vi "SYST_PRES.vi"(0 "VISA IN":refnum<visa-resource-name>, 5 "error in":errorcluster) -> (14 "VISA Out":refnum<visa-resource-name>, 19 "error out":errorcluster)   [LabVIEW 2018, in "PNA-X.lvlib"] (continued)
OFF (or 0) - Does NOT include DC Offset correction. \nExamples SENS:CORR:EXT:AUTO:DCOF 1 \nsense2:correction:extension:auto:dcoffset off \nQuery Syntax SENSe<cnum>:CORRection:EXTension:AUTO:DCOFfset? \nReturn Type Boolean \nDefault OFF (0) \nSENSe<cnum>:CORRection:EXTension:AUTO:LOSS <bool> \n(Read-Write) Specifies whether or not to include loss correction as part of automatic port extension. \nLearn more about Loss Compensation in port extension. \nParameters \n<cnum> Any existing channel number. If unspecified, value is set to 1 \n<bool> ON (or 1) - Includes Loss correction. \nOFF (or 0) - Does NOT include Loss correction. \nExamples SENS:CORR:EXT:AUTO:LOSS 1 \nsense2:correction:extension:auto:loss off \nQuery Syntax SENSe<cnum>:CORRection:EXTension:AUTO:LOSS? \nReturn Type Boolean \nDefault OFF (0) \nSENSe<cnum>:CORRection:EXTension:AUTO:MEASure <char> \n1701\n\n(Write-only) Measures either an OPEN or SHORT standard. When this command is sent, the PNA \nacquires the measurement with which to set automatic port extensions. Learn more about which \nstandard to measure. \nParameters \n<cnum> Any existing channel number. If unspecified, value is set to 1 \n<char> Standard to be measured. Choose from: \nOPEN Measure OPEN standard \nSHORt Measure SHORT standard \nExamples SENS:CORR:EXT:AUTO:MEAS OPEN \nsense2:correction:extension:auto:measure short \nQuery Syntax Not Applicable \nDefault Not Applicable \nSENSe<cnum>:CORRection:EXTension:AUTO:PORT<n> <bool> \n(Read-Write) Enables and disables automatic port extensions on the specified port. \nParameters \n<cnum> Any existing channel number. If unspecified, value is set to 1 \n<n> PNA Port number to enable or disable for automatic port extensions. \n<bool> ON (or 1) - Enable \nOFF (or 0) - Disable \nExamples SENS:CORR:EXT:AUTO:PORT2 0 \nsense2:correction:extension:auto:port4 on \nQuery Syntax SENSe<cnum>:CORRection:EXTension:AUTO:PORT<n>? \nReturn Type Boolean \nDefault All ports ON (enabled) \nSENSe<cnum>:CORRection:EXTension:AUTO:RESet \n1702\n\n(Write-only) Clears old port extension delay and loss data in preparation for acquiring new data. Send \nthis command prior to sending a new series of SENS:CORR:EXT:AUTO:MEAS. If acquiring both \nOPEN and SHORT standards, do not send this command between those acquisitions. \nParameters \n<cnum> Any existing channel number. If unspecified, value is set to 1 \nExamples SENS:CORR:EXT:AUTO:RES \nsense2:correction:extension:auto:reset \nQuery Syntax Not Applicable \nDefault Not Applicable \nSENSe<cnum>:CORRection:EXTension:AUTO:STARt <value> \n(Read-Write) Set the start frequency for custom user span. Learn more about User Span. \nParameters \n<cnum> Any existing channel number. If unspecified, value is set to 1 \n<value> User span start value. Must be within the frequency range of the active channel \nand less than the value set by SENS:CORR:EXT:AUTO:STOP. \nExamples SENS:CORR:EXT:AUTO:STAR 1E9 \nsense2:correction:extension:auto:start 200e6 \nQuery Syntax SENSe<cnum>:CORRection:EXTension:AUTO:STARt <value>? \nReturn Type Numeric \nDefault Start frequency of the current active channel. \nSENSe<cnum>:CORRection:EXTension:AUTO:STOP <value> \n1703\n\n(Read-Write) Set the stop frequency for custom user span. Learn more about User Span. \nParameters \n<cnum> Any existing channel number. If unspecified, value is set to 1 \n<value> User span stop value. Must be within the frequency range of the active channel \nand greater than the value set by SENS:CORR:EXT:AUTO:STARt \nExamples SENS:CORR:EXT:AUTO:STOP 1E9 \nsense2:correction:extension:auto:stop 200e6 \nQuery Syntax SENSe<cnum>:CORRection:EXTension:AUTO:STOP <value>? \nReturn Type Numeric \nDefault Stop frequency of the current active channel. \nSENSe<cnum>:CORRection:EXTension:PORT<pnum>:FREQ<n> <value> \n(Read-Write) Sets and returns the frequency \"Use\" number (1|2) for the specified port number. \nLearn about Loss Compensation values. \nParameters \n<cnum> Any existing channel number. If unspecified, value is set to 1 \n<pnum> Port Number that will receive the freq/loss settings. If unspecified, value is set \nto 1. \n<n> Frequency \"Use\" number. Choose from 1 or 2. If unspecified, value is set to 1. \n<value> Frequency value. Choose a frequency within the frequency span of the PNA. \nExamples SENS:CORR:EXT:PORT1:FREQ1 10E9 \nsense2:correction:extension:port2:freq2:2E10 \nQuery Syntax SENSe<cnum>:CORRection:EXTension:PORT<pnum>:FREQ<n>? \nReturn Type Numeric \nDefault 1 GHz \nSENSe<cnum>:CORRection:EXTension:PORT<pnum>:INCLude<n>:STATe <bool> \n1704\n\n(Read-Write) Sets and returns the ON/OFF state for the use of the Loss and Freq values for the \nspecified port number. \nLearn about Loss Compensation values. \nNote: This command affects ALL measurements on the specified channel. \nParameters \n<cnum> Any existing channel number. If unspecified, value is set to 1 \n<pnum> Port Number that will receive the Freq/Loss settings. If unspecified, value is set to \n1. \n<n> Freq and Loss pair. Choose from 1 or 2. If unspecified, value is set to 1. \n<value> State of Freq and Loss values for port extension. \n0 or OFF Specified Freq and Loss values are OFF \n1 or ON Specified Freq and Loss values are ON \nExamples SENS:CORR:EXT:PORT:INCL 0 \nsense2:correction:extension:port2:include:state on \nQuery Syntax SENSe<cnum>:CORRection:EXTension:PORT<pnum>:INCLude:STATe? \nReturn Type Boolean \nDefault OFF \nSENSe<cnum>:CORRection:EXTension:PORT<pnum>:LDC <value> \n(Read-Write) Sets and returns the Port Loss at DC value for the specified port number. \nLearn about Loss Compensation values. \nNote: This command affects ALL measurements on the specified channel. \nParameters \n<cnum> Any existing channel number. If unspecified, value is set to 1 \n<pnum> Port number to receive Loss value. If unspecified, value is set to 1. \n<value> Loss in dB. Choose a value between -90 and 90 \nExamples SENS:CORR:EXT:PORT:LDC 1.5 \nsense2:correction:extension:port2:ldc .1 \nQuery Syntax SENSe<cnum>:CORRection:EXTension:PORT<pnum>:LDC? \n1705\n\nReturn Type Numeric \nDefault 0 \nSENSe<cnum>:CORRection:EXTension:PORT<pnum>:LOSS<n> <value> \n(Read-Write) Sets and returns the Loss value for the specified port number. \nLearn about Loss Compensation values. \nNote: This command affects ALL measurements on the specified channel. \nParameters \n<cnum> Any existing channel number. If unspecified, value is set to 1 \n<pnum> Port Number that will receive the Freq/Loss settings. If unspecified, value is set \nto 1. \n<n> Loss \"Use\" number. Choose from 1 or 2. If unspecified, value is set to 1. \n<value> Loss in dB. Choose a value between -90 and 90 \nExamples SENS:CORR:EXT:PORT:LOSS1 1 \nsense2:correction:extension:port2:loss2 .1 \nQuery Syntax SENSe<cnum>:CORRection:EXTension:PORT<pnum>:LOSS<n>? \nReturn Type Numeric \nDefault 0 \nSENSe<cnum>:CORRection:EXTension:PORT<pnum>[:TIME] <num> \n1706\n\n(Read-Write) Sets the extension value at the specified port. Must also set SENS:CORR:EXT ON. \nNote: This command affects ALL measurements on the specified channel. \nParameters \n<cnum> Any existing channel number. If unspecified, value is set to 1 \n<pnum> Port Number that will receive the extension. If unspecified, value is set to 1. \n<num> The port extension in seconds; may include suffix. Choose a number between: \n-1E18 and 1E18 \nExamples SENS:CORR:EXT:PORT 2MS \nsense2:correction:extension:port2 .00025 \nQuery Syntax SENSe<cnum>:CORRection:EXTension:PORT<pnum> [:TIME]? \nReturn Type Numeric \nDefault 0 \nSENSe<cnum>:CORRection:EXTension:RECeiver<Rnum>[:TIME] <num> OBSOLETE \n(Read-Write) This command has NO replacement and no longer works. \nSets the extension value at the specified receiver. Must also set SENS:CORR:EXT ON. \nNote: Before using this command you must select a measurement using CALC:PAR:SEL. You can \nselect one measurement for each channel. \nParameters \n<cnum> Any existing channel number. If unspecified, value is set to 1 \n<Rnum> Number of the receiver that will receive the extension. If unspecified, value is \nset to 1 \nChoose from: \n1 for Receiver A \n2 for Receiver B \n<num> The electrical length in seconds; may include suffix. Choose a number \nbetween: \n-10 and 10 \nExamples SENS:CORR:EXT:REC 2MS \nsense2:correction:extension:receiver2:time .00025 \nQuery Syntax SENSe<cnum>:CORRection:EXTension:RECeiver<Rnum> [:TIME]? \n1707\n\nReturn Type Numeric \nDefault 0 \nSENSe<cnum>:CORRection:EXTension[:STATe] <ON | OFF> \n(Read-Write) Turns port extensions ON or OFF. \nParameters \n<cnum> Any existing channel number. If unspecified, value is set to 1 \n<ON | OFF> ON (or 1) - turns port extensions ON. \nOFF (or 0) - turns port extensions is OFF. \nExamples SENS:CORR:EXT ON \nsense2:correction:extension:state off \nQuery Syntax SENSe<cnum>:CORRection:EXTension[:STATe]? \nReturn Type Boolean (1 = ON, 0 = OFF) \nDefault OFF \n1708\n\nSense:Correction:Collect:Session Commands \nThe commands in this topic are common to perform both SMC and VMC calibrations. A calibration \nsession is a term used to describe an instance of a SMC or VMC calibration. For more commands, see \nSESS:SMC and SESS:VMC. \nCommands to read (STEP?) and describe (DESC?) each step are provided to facilitate a remote user \ninterface. \nTo perform a NON - SMC or VMC calibration, use either Guided or Mechanical SCPI commands. \nClick on a blue keyword to view the command details. \nSee Also \nSCPI SMC and VMC calibration examples. \nLearn about SMC and VMC calibrations \nSynchronizing the PNA and Controller \nSCPI Command Tree \nSENSe<ch>:CORRection:COLLect:SESSion<n>:ACQuire <step> \n1709\n\n(Write only) Acquire a calibration measurement. \nParameters \n<ch> Any existing channel number. If unspecified, value is set to 1. \n<n> Session number. Choose from 1 to 16. \n<step> Step number to acquire. Use SENS:CORR:COLL:SESS:STEPS? to find the \nnumber of steps required for the calibration. \nExamples SENSe2:CORR:COLL:SESS6:ACQ 5 \nQuery Syntax Not Applicable \nDefault Not Applicable \nSENSe<ch>:CORRection:COLLect:SESSion<n>:CKIT:PORT<p>:CATalog? \n(Read only) Returns a list of cal kits that are compatible with the connector on port <p>. The port \nconnector type is set with SENS:CORR:COLL:SESS:CONN:PORT \nParameters \n<ch> Any existing channel number. If unspecified, value is set to 1. \n<n> Session number. Choose from 1 to 16. \n<p> Port number of connector to query for compatible cal kits. \nExamples SENS2:CORR:COLL:SESS6:CKIT:PORT2:CAT? \nReturn Type Comma separated string values \nDefault Not Applicable \nSENSe<ch>:CORRection:COLLect:SESSion<n>:CKIT:PORT<p>[:SELect] <calkit> \n1710\n\n(Read-Write) Set or return the Cal Kit for the specified port. Use \nSENS:CORR:COLL:SESS:CKIT:PORT:CAT? to list compatible Cal Kits. \nParameters \n<ch> Any existing channel number. If unspecified, value is set to 1 \n<n> Session number. Choose from 1 to 16. \n<p> Port number for which to set cal kit. \n<calkit> Cal Kit Name \nExamples SENS:CORR:COLL:SESS:CKIT:PORT:SEL 85091A \nSENS2:CORR:COLL:SESS6:CKIT:PORT2:SEL? \nQuery Syntax SENS<ch>:CORR:COLL:SESS<n>:CKIT:PORT<p>[:SEL] ? \nReturn Type String \nDefault Not Applicable \nSENSe<ch>:CORRection:COLLect:SESSion<n>:CONN:PORT<p>[:SEL] <conn> \n(Read-Write) Set the connector type and sex for the specified port number. Catalog valid connector \ntypes using SENS:CORR:COLL:GUID:CONN:CAT? \nParameters \n<ch> Any existing channel number. If unspecified, value is set to 1 \n<n> Session number. Choose from 1 to 16. \n<p> Port number for which to select a connector type. \n<conn> Name of the connector type \nExamples SENS2:CORR:COLL:SESS6:CONN:PORT1:SEL \"N Type\" \nQuery Syntax SENS<ch>:CORR:COLL:SESS<n>:CONN:PORT<p>[:SEL] ? \nReturn Type String \nDefault Not Applicable \nSENSe<ch>:CORRection:COLLect:SESSion<n>:DESC? <step> \n1711\n\n(Read-only) Returns the connection prompt for the step. List the number of steps in the calibration \nusing SENS:CORR:COLL:SESS:STEPS?. \nParameters \n<ch> Any existing channel number. If unspecified, value is set to 1 \n<n> Session number. Choose from 1 to 16. \n<step> Step number \nExamples SENS1:CORR:COLL:SESS6:DESC?3 \nReturn Type Numeric \nDefault Not Applicable \nSENSe<ch>:CORRection:COLLect:SESSion<n>:DONE \n(Write only) Ends the calibration sessions. Use SAVE? to calculate error terms and save the CalSet. \nParameters \n<ch> Any existing channel number. If unspecified, value is set to 1 \n<n> Session number. Choose from 1 to 16. \nExamples SENS1:CORR:COLL:SESS6:DONE \nQuery Syntax Not Applicable \nDefault Not Applicable \nSENSe<ch>:CORRection:COLLect:SESSion<n>:INITiate <string> \n1712\n\n(Write only) Initiates an SMC or VMC calibration session. Use the session number for subsequent \nSMC or VMC commands. \nParameters \n<ch> Any existing channel number. If unspecified, value is set to 1 \n<n> Session number. Choose from 1 to 16. If the session number already exists it \nwill be terminated and a new session initiated. \n<string> Name of the calibration. Choose from: \n\"VMC\" or \"VectorMixerCal.VMCType\" \n\"SMC\" or \"ScalarMixerCal.SMCType\" \nExamples SENS1:CORR:COLL:SESS6:INITiate \"VectorMixerCal.VMCType\" \nQuery Syntax Not Applicable \nDefault Not Applicable \nSENSe<ch>:CORRection:COLLect:SESSion<n>:SAVE? \n(Read only) Finish the SMC or VMC calibration, compute error terms, populate and save the CalSet, \nand return the GUID of the Cal Set. \nNote: The destination (Cal Register or User Cal Set) is determined by the setting of the \nSENS:CORR:PREFerence:CSET:SAVE command. \nParameters \n<ch> Any existing channel number. If unspecified, value is set to 1 \n<n> Session number. Choose from 1 to 16. \nExamples SENS1:CORR:COLL:SESS6:SAVE? \nReturn Type String specifying the GUID of the CalSet produced by this session. \nDefault Not Applicable \nSENSe<ch>:CORRection:COLLect:SESSion<n>:STEPs? \n1713\n\n(Read-only) Returns the number of steps required by the Calibration. \nTo ensure this query always completes successfully, first send the write command: \nSENS:CORR:COLL:SESS:STEP, then send the query. \nParameters \n<ch> Any existing channel number. If unspecified, value is set to 1 \n<n> Session number. Choose from 1 to 16. \nExamples SENS1:CORR:COLL:SESS6:STEPs? \nReturn Type Numeric \nDefault Not Applicable \n1714\n\nSense:Correction:Collect:Session:SMC Commands \nPerforms scalar (SMC) calibration on a frequency converting device. \nClick on a blue keyword to view the command details. \nSee Also \nExample Programs \nLearn about FCA Calibrations \nSynchronizing the PNA and Controller \nSCPI Command Tree \nNOTE: To configure a power meter and sensor see SOURce:POWer: commands. \nSENSe<ch>:CORRection:COLLect:SESSion<n >:SMC:ECAL:CHARacteriza <mod> ,<char> \n1715\n\n(Read-Write) Specifies the ECal module and characterization to be used for the SMC calibration. \nParameters \n<ch> Any existing channel number. If unspecified, value is set to 1 \n<n> Session number. Choose from 1 to 16. Learn about Cal sessions. \n<mod> 1 - Electronic Calibration Module \n<char> Specifies which characterization within the ECal module from which to read \nthe confidence data. \n0 Factory characterization (data that was stored in the ECal module by \nAgilent). Default if not specified. \n1 User characterization #1 \n2 User characterization #2 \n3 User characterization #3 \n4 User characterization #4 \n5 User characterization #5 \nExamples SENS:CORR:COLL:SESS:SMC:ECAL:CHAR 1,2 \nQuery Syntax SENS:CORR:COLL:SESS:SMC:ECAL:CHAR? \nReturn Type Numeric \nDefault 1,0 \nSENSe<ch>:CORRection:COLLect:SESSion<n> :SMC:FSIMulator:NETWork<x>:MODE \n<char> \n1716\n\n(Read-Write) Allows you to embed (add) or de-embed (remove) circuit network effects on the input \nand output of your mixer measurement. Learn more. \nParameters \n<ch> Any existing channel number. If unspecified, value is set to 1 \n<n> Session number. Choose from 1 to 16. Learn about Cal sessions. \n<x> Apply network to input or output of mixer. Choose from: \n1 - Input of mixer \n2 - Output of mixer \n<char> Choose from: \nNONE - Do nothing with effects of S2P file. \nEMBed - Add effects of S2P file from the measurement results. \nDEEMbed - Remove effects of S2P file from the measurement results. \nExamples SENS:CORR:COLL:SESS:SMC:FSIM:NETW1:MODE EMB \nQuery Syntax SENS<ch>:CORRection:COLLect:SESSion<n> \n:SMC:FSIMulator:NETWork<x>:MODE? \nReturn Type Character \nDefault NONE \nSENSe<ch>:CORRection:COLLect:SESSion<n> :SMC:FSIMulator:NETWork<x>:FILename \n<string> \n1717\n\n(Read-Write) Specifies the S2P filename to embed or de-embed on the input or output of your mixer \nmeasurement. Learn more. \nParameters \n<ch> Any existing channel number. If unspecified, value is set to 1 \n<n> Session number. Choose from 1 to 16. Learn about Cal sessions. \n<x> Apply network to input or output of mixer. Choose from: \n1 - Input of mixer \n2 - Output of mixer \n<string> Filename of the S2P used for embedding or de-embedding. Use the full path \nname, file name, and .S2P suffix, enclosed in quotes. \nExamples SENS:CORR:COLL:SESS:SMC:FSIM:NETW1:FIL \"C:\\Program \nFiles\\Agilent\\Network Analyzer\\Documents\\WaveguideAdapt.S2P\" \nQuery Syntax SENS<ch>:CORRection:COLLect:SESSion<n> \n:SMC:FSIMulator:NETWork<x>:FILename? \nReturn Type String \nDefault Not Applicable \nSENSe<ch>:CORRection:COLLect:SESSion<n>:SMC:PWRCal:SRCPort <string> Obsolete \n(Read-Write) Specifies which port to calibrate. \nNote: Beginning with Rev 6.0, this command is no longer necessary. Learn more. Because of \nimproved calibration techniques, Both is always selected although a power meter measurement is \nperformed only on port 1. \nParameters \n<ch> Any existing channel number. If unspecified, value is set to 1 \n<n> Session number. Choose from 1 to 16. Learn about Cal sessions. \n<char> '1' Source port 1 (SMC forward direction) \n'2' Source port 2 (SMC reverse direction \n'BOTH' (both forward and reverse directions) \nExamples SENS:CORR:COLL:SESS:SMC:PWRC:SRCP 'both' \nSENSe2:CORRection:COLLection:SESSion6:SMC:PWRCal:SRCPort '2' \nQuery Syntax SENS:CORR:COLL:SESS:SMC:PWRC:SRCP? \n1718\n\nReturn Type String \nDefault 1 \nSENSe<ch>:CORRection:COLLect:SESSion<n>:SMC:TWOPort:ECAL:ORIentation[:STATe] \n<bool> \n(Read-Write) Sets ECAL Auto-Orientation ON or OFF. If setting auto-orientation OFF, you must \nmanually specify the orientation of the ECAL module with \nSENS:CORR:COLL:SESS:SMC:TWOP:ECAL:PORTmap. \nParameters \n<ch> Any existing channel number. If unspecified, value is set to 1 \n<n> Session number. Choose from 1 to 16. Learn about Cal sessions. \n<bool> 0 = Orientation OFF \n1 = Orientation ON \nExamples SENS:CORR:COLL:SESS:SMC:TWOP:ECAL:ORI 1 \nQuery Syntax SENS:CORR:COLL:SESS:SMC:TWOP:ECAL:ORI? \nReturn Type Boolean \nDefault 1 \nSENSe<ch>:CORRection:COLLect:SESSion<n>:SMC:TWOPort:ECAL:PORTmap <mod>, \n<string> \n(Read-Write) Specifies the manual orientation (which ports of the module are connected to which \nports of the PNA) when auto-orientation is OFF. \nParameters \n<ch> Any existing channel number. If unspecified, value is set to 1 \n<n> Session number. Choose from 1 to 16. Learn about Cal sessions. \n<mod> 1 - Electronic Calibration Module \n<string> Format in the following manner: \nAw,Bx,Cy,Dz \nwhere\nA, B, C, and D are literal ports on the ECAL module \n1719\n\nw,x,y, and z are substituted for PNA port numbers to which the ECAL module port \nis connected. \nPorts of the module which are not used are omitted from the string. \nFor example, on a 4-port ECal module with \nport A connected to PNA port 2 \nport B connected to PNA port 3 \nport C not connected \nport D connected to PNA port 1 \nthe string would be: A2,B3,D1 \nIf either the receive port or source port (or load port for 2-port cal) of the \nCALC:PAR:SELected measurement is not in this string and orientation is OFF, \nan attempt to perform an ECal calibration will fail. \nExamples SENS:CORR:COLL:SESS:SMC:TWOP:ECAL:PORTmap 1,'A1,B2' \nQuery Syntax SENS:CORR:COLL:SESS:SMC:TWOP:ECAL:PORTmap? \nReturn Type String \nDefault \"A1,B2\" \nSENSe<ch>:CORRection:COLLect:SESSion<n >:SMC:TWOPort:METHod <string> \n1720\n\n(Read-Write) Specifies the guided ECal method for performing the thru portion of the calibration. \nParameters \n<ch> Any existing channel number. If unspecified, value is set to 1 \n<n> Session number. Choose from 1 to 16. Learn about Cal sessions. \n<string> ECAL Method: Choose from: \n'DEFAULT' - Default \n'ADAP' - Adapter removal \n'FLUSH' - Flush Through \n'UNKN' - Unknown Thru \nExamples SENS:CORR:COLL:SESS:SMC:TWOPort:METH 'default' \nQuery Syntax SENS:CORR:COLL:SESS:SMC:TWOPort:METH? \nReturn Type String \nDefault DEFAULT \nSENSe<ch>:CORRection:COLLect:SESSion<n >:SMC:TWOPort:OMITisolat <bool> \n(Read-Write) Select to omit or perform the isolation portion of the ECAL. \nParameters \n<ch> Any existing channel number. If unspecified, value is set to 1 \n<n> Session number. Choose from 1 to 16. Learn about Cal sessions. \n<bool> 1 - Omit isolation \n0 - Perform isolation \nExamples SENS:CORR:COLL:SESS:SMC:TWOPort:OMIT 1 \nQuery Syntax SENS:CORR:COLL:SMC:TWOPort:OMIT? \nReturn Type Boolean \nDefault 1 \nSENSe<ch>:CORRection:COLLect:SESSion<n >:SMC:TWOPort:OPTion <string> \n1721\n\n(Read-Write) Sets the SMC calibration to ECAL or MECHanical \nParameters \n<ch> Any existing channel number. If unspecified, value is set to 1 \n<n> Session number. Choose from 1 to 16. Learn about Cal sessions. \n<char> Choose from: \n'ECAL' Electronic Calibration Module \n'MECH' Mechanical Calibration Kit \nExamples SENS:CORR:COLL:SESS:SMC:TWOPort:OPTion 'ECAL' \nQuery Syntax SENS:CORR:COLL:SESS:SMC:TWOPort:OPTion? \nReturn Type String \nDefault ECAL \n1722\n\nSense:Correction:Collect:Session:VMC Commands \nPerforms a vector (VMC) calibration on a frequency converting device. \nClick on a blue keyword to view the command details. \nSee Also \nExample Programs \nLearn about VMC Calibration \nSynchronizing the PNA and Controller \nSENSe<ch>:CORRection:COLLect:SESSion<n> :VMC:FSIMulator:NETWork<x>:MODE \n<char> \n1723\n\n(Read-Write) Allows you to embed (add) or de-embed (remove) circuit network effects on the input \nand output of your mixer measurement. Learn more. \nParameters \n<ch> Any existing channel number. If unspecified, value is set to 1 \n<n> Session number. Choose from 1 to 16. Learn about Cal sessions. \n<x> Apply network to input or output of mixer. Choose from: \n1 - Input of mixer \n2 - Output of mixer \n<char> Choose from: \nNONE - Do nothing with effects of S2P file. \nEMBed - Add effects of S2P file from the measurement results. \nDEEMbed - Remove effects of S2P file from the measurement results. \nExamples SENS:CORR:COLL:SESS:VMC:FSIM:NETW1:MODE EMB \nQuery Syntax SENS<ch>:CORRection:COLLect:SESSion<n> \n:VMC:FSIMulator:NETWork<x>:MODE? \nReturn Type Character \nDefault NONE \nSENSe<ch>:CORRection:COLLect:SESSion<n> :VMC:FSIMulator:NETWork<x>:FILename \n<string> \n1724\n\n(Read-Write) Specifies the S2P filename to embed or de-embed on the input or output of your mixer \nmeasurement. Learn more. \nParameters \n<ch> Any existing channel number. If unspecified, value is set to 1 \n<n> Session number. Choose from 1 to 16. Learn about Cal sessions. \n<x> Apply network to input or output of mixer. Choose from: \n1 - Input of mixer \n2 - Output of mixer \n<string> Filename of the S2P used for embedding or de-embedding. Use the full path \nname, file name, and .S2P suffix, enclosed in quotes. \nExamples SENS:CORR:COLL:SESS:VMC:FSIM:NETW1:FIL \"C:\\Program \nFiles\\Agilent\\Network Analyzer\\Documents\\WaveguideAdapt.S2P\" \nQuery Syntax SENS<ch>:CORRection:COLLect:SESSion<n> \n:VMC:FSIMulator:NETWork<x>:FILename? \nReturn Type String \nDefault Not Applicable \nSENSe<ch>:CORRection:COLLect:SESSion<n> :VMC:MIXer:CHARacterize:CAL:FILename \n<string> \n(Read-Write) Specifies the .S2P filename used for mixer characterization. Use the \nVMC:MIXer:CHARacterize:CAL: OPTion command to recall the file for mixer characterization. \nOnce recalled, use this command to query the current filename or set a new filename. \nParameters \n<ch> Any existing channel number. If unspecified, value is set to 1 \n<n> Session number. Choose from 1 to 16. Learn about Cal sessions. \n<string> Filename of the S2P used for mixer characterization. Use the full path name, \nfile name, and .S2P suffix, enclosed in quotes. \nExamples SENS2:CORR:COLL:SESS4:VMC:MIXer:CHAR:CAL:FILE \"C:\\Program \nFiles\\Agilent\\Network Analyzer\\Documents\\MyMixer.S2P\" \nQuery Syntax SENS:CORR:COLL:SESS:VMC:MIX:CHAR:CAL:FIL? \nReturn Type String \nDefault C:\\Program Files\\Agilent\\Network Analyzer\\Documents\\default.s2p \n1725\n\nSENSe<ch>:CORRection:COLLect:SESSion<n> :VMC:MIXer:CHARacterize:CAL: OPTion \n<char> \n(Read-Write) Sets the mixer characterization method to ECal, Mechanical, or read from a file. \nParameters \n<ch> Any existing channel number. If unspecified, value is set to 1 \n<n> Session number. Choose from 1 to 16. Learn about Cal sessions. \n<char> ECAL - Electronic Calibration Module \nMECH - Mechanical Calibration Kit \nFILE, <filename> - Retrieve a mixer characterization file. Also specify the \nfilename of the S2P used for mixer characterization. Use the full path name, \nfile name, and .S2P suffix. Use the VMC:CHARacterize:CAL:FILename \ncommand to query the filename.. \nExamples SENS:CORR:COLL:SESS:VMC:MIX:CHAR:CAL:OPT ECAL \nSENS2:CORR:COLL:SESS6:VMC:MIXer:CHAR:CAL:OPTion FILE, \nMyMixerFile.mxr \nQuery Syntax SENS:CORR:COLL:SESS:VMC:MIX:CHAR:CAL:OPT? \nReturn Type String \nDefault MECH \nSENSe<ch>:CORRection:COLLect:SESSion<n> :VMC:MIXer:CHARacterize:CAL: REVerse \n<bool> \n(Read-Write) Specifies the direction in which to characterize the calibration mixer. Learn more about \nthe calibration mixer. \nParameters \n<ch> Any existing channel number. If unspecified, value is set to 1 \n<n> Session number. Choose from 1 to 16. Learn about Cal sessions. \n<bool> False (0) - Characterize the calibration mixer in the SAME direction as that \nspecified in the mixer setup. \nTrue (1) - Characterize the calibration mixer in the REVERSE direction as that \nspecified in the mixer setup. \nExamples SENS:CORR:COLL:SESS:VMC:MIX:CHAR:CAL:REV 1 \n1726\n\nQuery Syntax SENS:CORR:COLL:SESS:VMC:MIX:CHAR:CAL:REV? \nReturn Type Boolean \nDefault False \nSENSe<ch>:CORRection:COLLect:SESSion<n > :VMC:MIXer:ECAL:CHARacteriza <mod> \n,<char> \n(Read-Write) Specifies the ECal module and characterization to be used for the mixer characterization \nportion of the calibration. \nParameters \n<ch> Any existing channel number. If unspecified, value is set to 1 \n<n> Session number. Choose from 1 to 16. Learn about Cal sessions. \n<mod> 1 - Electronic Calibration Module \n<char> Characterization number in the specified ECAL module. Choose from: \n0 Factory characterization (data that was stored in the ECal module by \nAgilent). Default if not specified. \n1 User characterization #1 \n2 User characterization #2 \n3 User characterization #3 \n4 User characterization #4 \n5 User characterization #5 \nExamples SENS:CORR:COLL:SESS:VMC:MIX:ECAL:CHAR 1,0 \nQuery Syntax SENS:CORR:COLL:SESS:VMC:MIX:ECAL:CHAR? \nReturn Type Numeric \nDefault 1,0 \nSENSe<ch>:CORRection:COLLect:SESSion<n> :VMC:MIXer:ECAL:PORTmap <mod>, \n<string> \n1727\n\n(Read-Write) Sets the port mapping for the mixer characterization with ECal. This command is \nrequired if SENS:CORR:COLL:SESS:VMC:MIX:CHAR:CAL:OPT ECAL is specified. \nParameters \n<ch> Any existing channel number. If unspecified, value is set to 1 \n<n> Session number. Choose from 1 to 16. Learn about Cal sessions. \n<mod> 1 - Electronic Calibration Module \n<string> Choose from: \n\"A1\" - ECAL module port A is connected to PNA port 1 \n\"B1\" - ECAL module port B is connected to PNA port 1 \nExamples SENS:CORR:COLL:SESS:VMC:MIX:ECAL:PORT? \nSENS2:CORR:COLL:SESS:VMC:MIXer:ECAL:PORTmap 1,\"A1\" \nQuery Syntax SENS:CORR:COLL:SESS:VMC:MIX:ECAL:PORTmap? \nReturn Type String \nDefault \"A1\" \nSENSe<ch>:CORRection:COLLect:SESSion<n>:VMC:OPERation <string> \n(Read-Write) Perform either full VMC calibration or mixer characterization only. \nParameters \n<ch> Any existing channel number. If unspecified, value is set to 1 \n<n> Session number. Choose from 1 to 16. Learn about Cal sessions. \n<char> 'CAL' - full calibration and mixer characterization \n'CHAR' - mixer characterization only (no reference mixer required) - Saves \nan .S2P file with the filename specified in \nSENS<ch>:CORR:COLL:SESSion<n >:VMC:CHARacterize:CAL:FILename \n<filename> . If none is specified, a filename is automatically generated and can \nbe queried using the filename command. \nExamples SENS:CORR:COLL:SESS:VMC:OPER 'CAL' \nQuery Syntax SENS:CORR:COLL:SESS:VMC:OPER? \nReturn Type String \nDefault CAL \n1728\n\nSENSe<ch>:CORRection:COLLect:SESSion<n> :VMC:TWOPort:ECAL:CHARacteriza <mod> \n,<char> \n(Read-Write) Specifies the ECal module and characterization to be used for the VMC calibration. \nParameters \n<ch> Any existing channel number. If unspecified, value is set to 1 \n<n> Session number. Choose from 1 to 16. Learn about Cal sessions. \n<mod> 1 - Electronic Calibration Module \n<char> Characterization number in the specified ECAL module. Choose from: \n0 Factory characterization (data that was stored in the ECal module by \nAgilent). Default if not specified. \n1 User characterization #1 \n2 User characterization #2 \n3 User characterization #3 \n4 User characterization #4 \n5 User characterization #5 \nExamples SENS:CORR:COLL:SESS:VMC:TWOP:ECAL:CHAR 1,1 \nQuery Syntax SENS:CORR:COLL:SESS:VMC:TWOP:ECAL:CHAR? \nReturn Type Integer \nDefault 1,0 \nSENSe<ch>:CORRection:COLLect:SESSion<n> :VMC:TWOPort:ECAL:ORIentation[:STATe] \n<bool> \n1729\n\n(Read-Write) Sets ECAL orientation for the VMC ECal. \nParameters \n<ch> Any existing channel number. If unspecified, value is set to 1 \n<n> Session number. Choose from 1 to 16. Learn about Cal sessions. \n<bool> 1 = ON \n0 = OFF \nExamples SENS:CORR:COLL:SESS:VMC:TWOP:ECAL:ORI 1 \nQuery Syntax SENS:CORR:COLL:SESSion:VMC:TWOPort:ECAL:ORIentation[:STATe]? \nReturn Type Integer \nDefault ON \nSENSe<ch>:CORRection:COLLect:SESSion<n> :VMC:TWOPort:ECAL:PORTmap <mod>, \n<string> \n(Read-Write) Specifies the manual orientation (which ports of the module are connected to which \nports of the PNA) when orientation is turned off. \nParameters \n<ch> Any existing channel number. If unspecified, value is set to 1 \n<n> Session number. Choose from 1 to 16. Learn about Cal sessions. \n<mod> 1 - Electronic Calibration Module \n<string> Port Map, formatted in the following manner: \nAw,Bx,Cy,Dz \nwhere: \nA, B, C, and D are literal ports on the ECAL module. \nw,x,y, z are substituted for PNA port numbers to which the ECAL module port is \nconnected. \nPorts of the module which are not used are omitted from the string. \nFor example, on a 4-port ECal module with: \nport A connected to PNA port 2 \n1730\n\nport B connected to PNA port 3 \nport C not connected \nport D connected to PNA port 1 \nthe string would be: A2,B3,D1 \nIf either the receive port or source port (or load port for 2-port cal) of the \nmeasurement is not in this string and orientation is OFF, an attempt to perform \nan ECal will fail. \nExamples SENS:CORR:COLL:SESS:VMC:TWOP:ECAL:PORTmap 1,\"A2,B1\" \nQuery Syntax SENS:CORR:COLL:SESS:VMC:TWOP:ECAL:PORTmap? \nReturn Type string \nDefault \"A1,B2\" \nSENSe<ch>:CORRection:COLLect:SESSion<n> :VMC:TWOPort:METHod <string> \n(Read-Write) Specifies the guided ECal method for performing the thru portion of the calibration. \nParameters \n<ch> Any existing channel number. If unspecified, value is set to 1 \n<n> Session number. Choose from 1 to 16. Learn about Cal sessions. \n<char> 'DEFAULT' - Default \n'ADAP' - Adapter removal \n'FLUSH' - Flush Through \n'UNKN' - Unknown Thru \nExamples SENS:CORR:COLL:SESS:VMC:TWOP:METH 'ADAP' \nSENSe2:CORR:COLL:SESSion6:VMC:TWOPort:METHod 'FLUSH' \nQuery Syntax SENS:CORR:COLL:SESS:VMC:TWOP:METH? \nReturn Type String \nDefault DEFAULT \nSENSe<ch>:CORRection:COLLect:SESSion<n> :VMC:TWOPort:OMITisolat <bool> \n1731\n\n(Read-Write) Select to omit or perform the isolation portion of the ECAL. \nParameters \n<ch> Any existing channel number. If unspecified, value is set to 1 \n<n> Session number. Choose from 1 to 16. Learn about Cal sessions. \n<bool> 1 - omit isolation \n0 - perform isolation \nExamples SENS:CORR:COLL:SESS:VMC:TWOP:OMIT 1 \nQuery Syntax SENS:CORR:COLL:SESS:VMC:TWOP:OMIT? \nReturn Type Numeric \nDefault 1 \nSENSe<ch>:CORRection:COLLect:SESSion<n> :VMC:TWOPort:OPTion <string> \n(Read-Write) Sets the 2-port calibration option to ECAL or MECHanical \nParameters \n<ch> Any existing channel number. If unspecified, value is set to 1 \n<n> Session number. Choose from 1 to 16. Learn about Cal sessions. \n<char> \nChoose from: \n'ECAL' Electronic Calibration Module \n'MECH' Mechanical Calibration Kit \nExamples SENS:CORR:COLL:SESS:VMC:TWOP:OPT 'MECH' \nSENSe2:CORR:COLL:SESSion6:VMC:TWOPort:OPTion 'ECAL' \nQuery Syntax SENS:CORR:COLL:SESS:VMC:TWOP:OPT? \nReturn Type String \nDefault \"MECH\" \n1732\n\nSense:Couple Commands \nClick on a blue keyword to view the command details. \nSee Also \nExample Programs \nSynchronizing the PNA and Controller \nSCPI Command Tree \nSENSe<cnum>:COUPle <ALL | NONE> \n(Read-Write) Sets the sweep mode as Chopped or Alternate. \nLearn about Alternate Sweep \nParameters \n<cnum> Any existing channel number; if unspecified, value is set to 1. \n<ALL | NONE> ALL - Sweep mode set to Chopped - reflection and transmission measured on \nthe same sweep. \nNONE - Sweep mode set to Alternate - reflection and transmission measured \non separate sweeps. Improves Mixer bounce and Isolation measurements. \nIncreases sweep time \nExamples SENS:COUP ALL \nsense2:couple none \nQuery Syntax SENSe<cnum>:COUPle? \nReturn Type Character \nDefault ALL \nSENSe<cnum>:COUPle:PARameter[:STATe] <bool> \n1733\n\n(Read-Write) Turns ON and OFF Time Domain Trace Coupling. All of the measurements in the \nspecified channel are coupled. \nTo select Transform parameters to couple, use CALC:TRAN:COUP:PAR \nTo select Gating parameters to couple, use CALC:FILT:COUP:PAR \nLearn more about Time Domain Trace Coupling. \nParameters \n<cnum> Any existing channel number; if unspecified, value is set to 1. \n<bool> ON (or 1) - Turns ON Time Domain Trace Coupling. \nOFF (or 0) - Turns OFF Time Domain Trace Coupling. \nExamples SENS:COUP:PAR 0 \nsense2:couple:parameter:state on \nQuery Syntax SENSe<cnum>:COUPle:PARameter[:STATe]? \nReturn Type Boolean \nDefault ON (or 1) \n1734\n\nSense:FOM (Frequency Offset) Commands \nControls the frequency offset settings which cause stimulus and response frequencies to be different. \nNote: These commands supersede previous FOM commands. Although the old commands will continue to work, \nthey can NOT be mixed with these new commands. \nClick on a blue keyword to view the command details. \nSee Also \nExample Programs \nLearn about Frequency Offset \nSynchronizing the PNA and Controller \nSCPI Command Tree \nSENSe<cnum>:FOM[:STATe] <bool> \n1735\n\n(Read-Write) Turns Frequency Offset ON and OFF. Frequency offset settings are not enabled until this setting is \nON. \nSend this command (FOM ON) AFTER sending other FOM settings to avoid 'out-or-range' errors. \nParameters \n<cnum> Any existing channel number; if unspecified, value is set to 1. \n<bool> ON (or 1) - turns FOM ON. \nOFF (or 0) - turns FOM OFF. \nExamples SENS:FOM 1 \nsense2:fom:state on \nQuery Syntax SENSe<cnum>:FOM:STATe? \nReturn Type Boolean \nDefault OFF \nSENSe<cnum>:FOM:CATalog? \n(Read-only) Returns a comma-separated list of available range names in the PNA. \nParameters \n<cnum> Any existing channel number; if unspecified, value is set to 1. \nExamples SENS:FOM:CAT? \n'returns \n\"Primary, Source, Receivers\" \nReturn Type String \nDefault Not Applicable \nSENSe<cnum>:FOM:COUNt? \n1736\n\n(Read-only) Returns the number of valid ranges in the PNA. \nParameters \n<cnum> Any existing channel number; if unspecified, value is set to 1. \nExamples SENS:FOM:COUN? \nsense2:fom:count? \nQuery Syntax SENSe<cnum>:FOM:COUNt? \nReturn Type Numeric \nDefault Not Applicable \nSENSe<cnum>:FOM:DISPlay:SELect <string> \n(Read-Write) Select the range to be displayed on the PNA x-axis. All traces in the channel have this same x-axis \nscaling. \nParameters \n<cnum> Any existing channel number; if unspecified, value is set to 1. \n<string> Range name. Case insensitive. Use SENSe:FOM:CAT? to see a list of available \nfrequency range names. \nExamples SENS:FOM:DISPlay:SELect \"source2\" \nsense2:fom:display:select \"source\" \nQuery Syntax SENSe<cnum>:FOM:DISPlay:SELect? \nReturn Type String \nDefault Receivers \nSENSe<cnum>:FOM:RNUM? <string> \n1737\n\n(Read-only) Returns the number of a specified range name. \nThe FOM range items are typically numbered as follows: \nPrimary 1. \nSource 2. \nReceivers 3. \nSource2 (if present) 4. \nParameters \n<cnum> Any existing channel number; if unspecified, value is set to 1. \n<string> Range name for which a number is being queried. Case insensitive. Use \nSENSe:FOM:CAT? to see a list of available range names. \nExamples SENS:FOM:RNUM? \"receivers\" \nsense2:fom:rnum? \"Source2\" \nReturn Type Numeric \nDefault Not Applicable \nSENSe<cnum>:FOM:RANGe<n>:COUPled <bool> \n(Read-Write) Sets and returns the state of coupling (ON or OFF) of the specified range to the primary range. \nParameters \n<cnum> Any existing channel number; if unspecified, value is set to 1. \n<n> Range number to couple to primary range. An error is returned when attempting to \ncouple to the Primary range (1). \n<bool> ON (or 1) - Couple range to primary range. \nOFF (or 0) - Do NOT couple to primary range. \nExamples SENS:FOM:RANG:COUP 1 \nsense2:fom:range2:coupled 0 \nQuery Syntax SENSe<cnum>:FOM:RANGe<n>:COUPled? \nReturn Type Boolean \nDefault ON (or 1) Coupled \n1738\n\nSENSe<cnum>:FOM:RANGe<n>:FREQuency:CW <num> \n(Read-Write) Sets and returns the CW frequency. \nThis setting is valid for the primary range, or if the specified range is already uncoupled from the primary range \nand if the sweep type is CW. \nParameters \n<cnum> Any existing channel number; if unspecified, value is set to 1. \n<n> Range number. If unspecified, value is set to 1. \n<num> CW frequency value in Hz. Choose any frequency within the range of the PNA. \nExamples SENS:FOM:RANG:FREQ:CW 1e9 \nsense2:fom:range2:frequency:cw 10000000 \nQuery Syntax SENSe<cnum>:FOM:RANGe:<n>:FREQuency:CW? \nReturn Type Numeric \nDefault Center frequency of the PNA. \nSENSe<cnum>:FOM:RANGe<n>:FREQuency:DIVisor <num> \n(Read-Write) Sets and returns the divisor value. \nThis setting is valid only if the specified range is coupled to the primary range. \nParameters \n<cnum> Any existing channel number; if unspecified, value is set to 1. \n<n> Range number. If unspecified, value is set to 1. \n<num> Divisor value (unitless). \nExamples SENS:FOM:RANG:FREQ:DIV 3 \nsense2:fom:range2:frequency:divisor 0 \nQuery Syntax SENSe<cnum>:FOM:RANGe<n>:FREQuency:DIVisor? \nReturn Type Numeric \nDefault 1 \n1739\n\nSENSe<cnum>:FOM:RANGe<n>:FREQuency:MULTiplier <num> \n(Read-Write) Sets and returns the multiplier value to be used when coupling this range to the primary range. \nThis setting is valid only if the specified range is coupled to the primary range. \nParameters \n<cnum> Any existing channel number; if unspecified, value is set to 1. \n<n> Range number. If unspecified, value is set to 1. \n<num> Multiplier value. (Unitless) \nExamples SENS:FOM:RANG:FREQ:MULT 1 \nsense2:fom:range2:frequency:multiplier 2 \nQuery Syntax SENSe<cnum>:FOM:RANGe<n>:FREQuency:MULTplier? \nReturn Type Numeric \nDefault 1 \nSENSe<cnum>:FOM:RANGe<n>:FREQuency:OFFSet <num> \n(Read-Write) Sets and returns the offset value to be used when coupling this range to the primary range. Learn \nmore about offset value. \nThis setting is valid only if the specified range is coupled to the primary range. \nParameters \n<cnum> Any existing channel number; if unspecified, value is set to 1. \n<n> Range number. If unspecified, value is set to 1. \n<num> Offset value. (Unitless) \nExamples SENS:FOM:RANG:FREQ:OFFS 1E9 \nsense2:fom:range2:frequency:offset 10000000 \nQuery Syntax SENSe<cnum>:FOM:RANGe<n>:FREQuency:OFFSet? \nReturn Type Numeric \nDefault 0 \nSENSe<cnum>:FOM:RANGe<n>:FREQuency:STARt <num> \n1740\n\n(Read-Write) Sets and returns the Start value of frequency range. Also specify Stop frequency. \nThis setting is valid for the primary range, or if the specified range is already uncoupled from the primary range \nand if the sweep type is LOG or LINear. \nParameters \n<cnum> Any existing channel number; if unspecified, value is set to 1. \n<n> Range number. If unspecified, value is set to 1. \n<num> Start value in Hz. Choose any frequency within the range of the PNA. \nExamples SENS:FOM:RANG:FREQ:STAR 1GHz \nsense2:fom:range2:frequency:start 100000000 \nQuery Syntax SENSe<cnum>:FOM:RANGe<n>:FREQuency:STARt? \nReturn Type Numeric \nDefault Minimum frequency of the PNA. \nSENSe<cnum>:FOM:RANGe<n>:FREQuency:STOP <num> \n(Read-Write) Sets and returns the Stop value of frequency range. Also specify Start frequency. \nThis setting is valid for the primary range, or if the specified range is already uncoupled from the primary range \nand if the sweep type is LOG or LINear. \nParameters \n<cnum> Any existing channel number; if unspecified, value is set to 1. \n<n> Range number. If unspecified, value is set to 1. \n<num> Stop value in Hz. Choose any frequency within the range of the PNA. \nExamples SENS:FOM:RANG:FREQ:STOP 1e12 \nsense2:fom:range2:frequency:stop 10000000000 \nQuery Syntax SENSe<cnum>:FOM:RANGe<n>:FREQuency:STOP? \nReturn Type Numeric \nDefault Maximum frequency of the PNA. \nSENSe<cnum>:FOM:RANGe<n>:NAME? \n1741\n\n(Read-only) Returns the name of range<n>. \nThe FOM range items are typically named as follows: \nPrimary 1. \nSource 2. \nReceivers 3. \nSource2 (if present) 4. \nParameters \n<cnum> Any existing channel number; if unspecified, value is set to 1. \n<n> Range number. If unspecified, value is set to 1. \nExamples SENS:FOM:RANG:NAME? \nsense2:fom:range2:name? \nReturn Type String \nDefault Not Applicable \nSENSe<cnum>:FOM:RANGe<n>:SWEep:TYPE <char> \n(Read-Write) Sets and returns the sweep type to be used with the specified range. \nThis setting is valid only if the specified range is already uncoupled from the primary range. \nLearn about Unsupported Sweep Type combinations. \nParameters \n<cnum> Any existing channel number; if unspecified, value is set to 1. \n<n> Range number. If unspecified, value is set to 1. \n<char> Sweep type. Choose from: \nCW - Also specify CW frequency. \nLINear - Also specify frequency Start/Stop or Center/Span \nLOG - Also specify frequency Start/Stop or Center/Span \nPOWer - Also specify power Start/Stop or Center/Span \nSEGMent - Also specify segment sweep settings. \n1742\n\nExamples SENS:FOM:RANG:SWE:TYPE LOG \nsense2:fom:range2:sweep:type linear: \nQuery Syntax SENSe<cnum>:FOM:RANGe<n>:SWEep:TYPE? \nReturn Type Character \nDefault Linear \nLast Modified: \n8-Mar-2007 MQX New topic \n1743\n\nSense:Frequency Commands \nSets the frequency sweep functions of the analyzer. \nClick on a blue keyword to view the command details. \nSee Also \nExample using some of these commands. \nLearn about Frequency Sweep \nSynchronizing the PNA and Controller \nSCPI Command Tree \nNote: All of the commands in this block will accept MIN or MAX instead of a numeric parameter. \nAlso, kHZ, MHz, and GHz are accepted as suffixes/units. \nSee SCPI Syntax for more information. \nSENSe<cnum>:FREQuency:CENTer <num> \n(Read-Write) Sets the center frequency of the analyzer. \nParameters \n<cnum> Any existing channel number. If unspecified, value is set to 1 \n<num> Center frequency. Choose any number between the minimum and maximum \nfrequency limits of the analyzer. Units are Hz. \nSee Note \nExamples SENS:FREQ:CENT 1000000 \nsense2:frequency:center 1mhz \nsense2:frequency:center 1e6 \nQuery Syntax SENSe<cnum>:FREQuency:CENTer? \nReturn Type Numeric \nDefault Center of the analyzer's frequency span \n1744\n\nSENSe<cnum>:FREQuency[:CW |:FIXed] <num> \n(Read-Write) Sets the Continuous Wave (or Fixed) frequency. Must also send SENS:SWEEP:TYPE \nCW to put the analyzer into CW sweep mode. \nParameters \n<cnum> Any existing channel number. If unspecified, value is set to 1 \n<num> CW frequency. Choose any number between the minimum and maximum \nfrequency limits of the analyzer. Units are Hz. \nSee Note \nExamples SENS:FREQ 1000000 \nSENS:FREQ:CW MIN \nsense2:frequency:fixed 1mhz \nQuery Syntax SENSe<cnum>:FREQuency[:CW | :FIXed]? \nReturn Type Numeric \nDefault 1 GHz \nSENSe<cnum>:FREQuency:SPAN <num> \n(Read-Write) Sets the frequency span of the analyzer. \nParameters \n<cnum> Any existing channel number. If unspecified, value is set to 1 \n<num> Frequency span. Choose any number between: \n0 (minimum) and the maximum frequency span of the analyzer. \nUnits are Hz \nSee Note \nExamples SENS:FREQ:SPAN 1000000 \nsense2:frequency:span max \nQuery Syntax SENSe<cnum>:FREQuency:SPAN? \nReturn Type Numeric \nDefault Maximum frequency span of the analyzer \nSENSe<cnum>:FREQuency:STARt <num> \n1745\n\n(Read-Write) Sets the start frequency of the analyzer. \nParameters \n<cnum> Any existing channel number. If unspecified, value is set to 1 \n<num> Start frequency. Choose any number between the MIN and MAX frequency \nlimits of the analyzer. Units are Hz \nIf FREQ:START is set greater than FREQ:STOP, then STOP is set equal to \nSTART. \nSee Note \nExamples SENS:FREQ:STAR 1000000 \nsense2:frequency:start MIN \nQuery Syntax SENSe<cnum>:FREQuency:STARt? \nIf Sweep type is segment, this query returns the start frequency of the first \nsegment. \nReturn Type Numeric \nDefault Minimum frequency of the analyzer \nSENSe<cnum>:FREQuency:STOP <num> \n(Read-Write) Sets the stop frequency of the analyzer. \nParameters \n<cnum> Any existing channel number. If unspecified, value is set to 1 \n<num> Stop frequency. Choose any number between: \nthe minimum and maximum frequency limits of the analyzer. Units are Hz \nIf FREQ:STOP is set less than FREQ:START, then START will be set equal to \nSTOP. \nSee Note \nExamples SENS:FREQ:STOP 1000000 \nsense2:frequency:stop max \nQuery Syntax SENSe<cnum>:FREQuency:STOP? \nIf Sweep type is segment, this query returns the stop frequency of the last segment. \nReturn Type Numeric \nDefault Maximum frequency of the analyzer \n1746\n\n1747\n\nSense:IF Commands \nControls the IF source and gain settings for use with the E836x H11 Option. \nSee IF/DSP and Pulse commands for the PNA-X. \nClick on a blue keyword to view the command details. \nSee IF Access User Interface Settings \nSynchronizing the PNA and Controller \nSCPI Command Tree \nSENSe<cnum>:IF:FILTer:SAMPle:COUNt <num> \n(Read-Write) Sets and returns the number of taps in the IF filter. The IF filter sample count setting is \nonly used when SENSe:IF:FILTer:SAMPle:COUNt:MODE is set to MANUAL. Critical Note: \nParameters \n<cnum> Existing channel number to manipulate. If unspecified, <cnum> is set to 1. \n<num> An integer value. (MIN and MAX return the minimum and maximum allowed values, \nrespectively.) \nExamples SENS:IF:FILT:SAMP:COUN 40 \nsense2:if:filter:sample:count maximum \nQuery Syntax SENS:IF:FILTer:SAMPle:COUNt? \nReturn Type Numeric \nDefault Instrument dependent. \nSENSe<cnum>:IF:FILTer:SAMPle:COUNt:MODE <char> \n1748\n\n(Read-Write) Sets and returns the IF filter sample count mode to the specified value. When in \nMANUAL mode, the value specified for the IF Filter sample count is used as the number of taps in the \nIF filter. Critical Note: \nParameters \n<cnum> Existing channel number to manipulate. If unspecified, <cnum> is set to 1. \n<char> Choose either AUTO or MANUAL. \nExamples SENS:IF:FILT:SAMP:COUN:MODE MANUAL \nsense2:if:filter:sample:count:mode AUTO \nQuery Syntax SENS:IF:FILTer:SAMPle:COUNt:MODE? \nReturn Type Character \nDefault AUTO \nSENSe<cnum>:IF:FILTer:SAMPle:PERiod <num> \n(Read-Write) Sets and returns the IF filter sample period. The IF filter sample period setting is only \nused by the instrument when the SENS:IF:FILT:SAMP:PER:MODE is set to MANUAL. Critical \nNote: \nParameters \n<cnum> Existing channel number to manipulate. If unspecified, <cnum> is set to 1. \n<num> Sample period. Choose from values returned from the \nSENS:IF:FILTer:SAMPle:PERiod:CAT? command. \nExamples SENS:IF:FILT:SAMP:PER 6 us \nsense2:if:filter:sample:period maximum \nQuery Syntax SENS:IF:FILTer:SAMPle:PERiod? \nReturn Type Numeric \nDefault Instrument dependent. \nSENSe<cnum>:IF:FILTer:SAMPle:PERiod:CATalog? \n(Read-Only) Returns the list of allowed IF filter sample periods for this instrument. Critical Note: \nParameters \n<cnum> Existing channel number to manipulate. If unspecified, <cnum> is set to 1. \nExamples SENS:IF:FILT:SAMP:PER:CAT? \nsense2:if:filter:sample:period:catalog? \nQuery Syntax SENS:IF:FILTer:SAMPle:PERiod:CATalog? \nReturn Type String \nDefault AUTO \n1749\n\nSENSe<cnum>:IF:FILTer:SAMPle:PERiod:MODE <char> \n(Read-Write) Sets and returns the IF filter sample period mode to the specified value. Critical Note: \nParameters \n<cnum> Existing channel number to manipulate. If unspecified, <cnum> is set to 1. \n<char> Sample period mode. Choose from AUTO or MANUAL. \nExamples SENS:IF:FILT:SAMP:PER:MODE MANUAL \nsense2:if:filter:sample:period:mode AUTO \nQuery Syntax SENS:IF:FILTer:SAMPle:PERiod:MODE? \nReturn Type Character \nDefault AUTO \nSENSe<cnum>:IF:GAIN:ALL[:STATe] <char> \n(Write only) Sets the gain state for ALL receivers to Auto or Manual. \nParameters \n<cnum> Existing channel number to manipulate. If unspecified, <cnum> is set to 1. \n<char> Choose from AUTO or MANUAL \nExamples SENS:IF:GAIN:ALL AUTO \nsense:if:gain:all:state manual \nQuery Syntax Not Applicable \nReturn Type Character \nDefault AUTO \nSENSe<cnum>:IF:GAIN:LEVel <id>, <level> \n1750\n\n(Read Write) Manually sets the gain level for the specified receiver. \nParameters \n<cnum> Existing channel number to manipulate. If unspecified, <cnum> is set to 1. \n<id> Choose from: 'A', 'B', 'R1', 'R2'. \nNote: The A and R1 receivers are always switched together. B and R2 are also \nalways switched together. For example, if you specify 'A', R1 will also be \nswitched. \n<level> Gain level. Choose from: \n0 - Lowest gain setting \n1\n2 - Highest gain setting \nExamples SENS:IF:GAIN:LEVel 'A', 1 \nQuery Syntax SENSe<cnum>:IF:GAIN:LEVel? <id> \nReturn Type Numeric \nDefault 0 \nSENSe<cnum>:IF:GAIN[:STATe]?, <id> \n(Read only) Returns the gain state for the specified receiver. Use SENS:IF:GAIN:ALL. to set the gain \nstate for all channels. \nParameters \n<cnum> Existing channel number to manipulate. If unspecified, <cnum> is set to 1. \n<id> Choose from: 'A', 'B', 'R1', 'R2'. \nNote: The A and R1 receivers are always switched together. B and R2 are also \nalways switched together. For example, if you specify 'A', R1 will also be \nswitched. \nExamples SENS:IF:GAIN? 'A' \nReturn Type Boolean \nDefault Not Applicable \n1751\n\nSENSe<cnum>:IF:GATE:STATe <boolean> \n(Read-Write) Sets or returns the IF filter gate state. \nParameters \n<cnum> Existing channel number to manipulate. If unspecified, <cnum> is set to 1. \n<boolean> Choose from ON or OFF \nExamples SENS:IF:FILT:GATE:STAT ON \nsense2:if:filter:gate:state 0 \nQuery Syntax SENS:IF:FILTer:SAMPle:COUNt:MODE? \nReturn Type Boolean \nDefault AUTO \nSENSe<cnum>:IF:SOURce:PATH <id>, <char> \n(Read Write) Sets the source path for the specified receiver. An error is returned if <id> is not valid, \nor if <char> is not valid for the specified <id>. \nParameters \n<cnum> Existing channel number to manipulate. If unspecified, <cnum> is set to 1. \n<id> Choose from: 'A', 'B', 'R1', 'R2' \nNote: The A and R1 receivers are always switched together. B and R2 are also \nalways switched together. For example, if you specify \"A\", R1 will also be \nswitched. \n<char> Choose from: \nNORMal - the PNA decides the appropriate IF input paths. \nEXTernal - always use the rear panel IF inputs. \nExamples SENS:IF:SOUR:PATH 'A', Ext \nQuery Syntax SENSe<cnum>:IF:SOURce:PATH? <id> \nReturn Type Character \nDefault Normal \n1752\n\nSense:IF Commands \nControls the IF filter for use with the PNA X. \nClick on a blue keyword to view the command details. \nSynchronizing the PNA and Controller \nSCPI Command Tree \nPNA-X DSP Block diagram \nAll of the Sense:IF commands, except the frequency commands, make settings related to the DSP section of the IF Path. \nSee the entire IF Path Configuration. \nNote: For any of the Filter \"Stage\" parameters to take effect, SENS:IF:FILT:AUTO must be set to OFF \n(MANUAL) and mode, and SENS:IF:FILT:CMOD must be set to OFF. \n1753\n\nCritical Note: These commands act on the selected measurement. You can select one measurement for \neach channel using Calc:Par:Select \nSENSe<cnum>:IF:FILTer:AUTO <bool> \n(Read-Write) Sets and returns whether the PNA configures the 3-stage digital filter settings or they \nwill be configured manually. When making manual settings, also send SENS:IF:FILT:CMOD OFF \nwhich routes the IF through the 3-stage filter. \nCritical Note \nParameters \n<cnum> Existing channel number. If unspecified, <cnum> is set to 1. \n<bool> (Boolean) \nON (or 1) - Automatic: PNA controls digital filter settings. \nOFF (or 0) - Manual: You control digital filter settings using other Sens:IF \ncommands. \nExamples SENS:IF:FILT:AUTO 1 \nsense2:if:filter:auto 0 \nQuery Syntax SENSe<cnum>:IF:FILTer:AUTO? \nReturn Type Boolean \nDefault ON \nSENSe:IF:FILTer:CMODe <bool> \n(Read-Write) Sets and returns the ADC capture mode modeled as a 2-pole switch in the above \ndiagram. The switch either bypasses or routes the IF through the 3-stage digital filter. \nCritical Note \nParameters \n<bool> (Boolean) \nON (or 1) - The digital filters are bypassed and the raw ADC readings are taken \ndirectly. A maximum of 4096 data points per sweep can be acquired. \nOFF (or 0) - The digital filters are used to process IF information. The filters \ncan be configured automatically or manually using SENS:IF:FILT:AUTO. \nExamples SENS:IF:FILT:CMOD 1 \nsense2:if:filter:cmode 0 \nQuery Syntax SENSe<cnum>:IF:FILTer:CMODe? \n1754\n\nReturn Type Boolean \nDefault OFF \nSENSe<cnum>:IF:FILTer:ERRors? \n(Read-only) Returns the error string associated with the digital filters. The return string has three fields \nseparated by commas: \"stage1 status, stage2 status, stage3 status\" \nEach of these fields can contain one or more of the following error codes: \nNO ERROR \n*NUMBER-OF-COEFFICIENTS - the number of coefficients is excessive for that filter-stage \n*COEFFICIENT VALUE - one or more coefficients are out of range for that filter-stage \n*SUM-OF-COEFFICIENTS - the sum of all coefficients is excessive for that filter-stage, \n*FREQUENCY - the frequency for Stage 1 is out of range (only applies stage1 field), \n*PARAMETER - one or more parameters are out of range (only applies to stage 3 field) \nCritical Note \nParameters \n<cnum> Existing channel number. If unspecified, <cnum> is set to 1. \nExamples SENS:IF:FILT:ERR? \n'example return strings\" \nNO ERROR, NO ERROR, NO ERROR \nindicates no errors, \n*SUM-OF-COEFFICIENTS, NO ERROR, NO ERROR \nindicates that the sum of all filter coefficients exceed the \nmaximum value for the Stage-1 filter, \n*COEFFICIENT *SUM-OF-COEFFICIENTS, NO ERROR, *PARAMETER \nindicates a problems with Stage 1 coefficients and a problem with \none or more of the parameters associated with the Stage 3 filter. \nReturn Type String \nDefault Not Applicable \nSENSe<cnum>:IF:FILTer:STAGE<n>:COEFficients <coef> \n1755\n\n(Read-Write) Sets and returns the digital filter coefficients of the specified stage. \nCritical Note \nParameters \n<cnum> Existing channel number. If unspecified, <cnum> is set to 1. \n<n> Stage number. Choose 1 or 2 \n<coef> An array of real numbers. Filter coefficients \nExamples SENS:IF:FILT:STAG2:COEF 0,0.1,0.7,0.7,0.1 \nsense2:if:filter:stage1:coefficients \nQuery Syntax SENSe<cnum>:IF:FILTer:STAGE<n>:COEFficients? \nExample SENS:IF:FILT:STAG2:COEF? \nsense2:if:filter:stage1:coefficients? \nReturn Type Numeric \nDefault Stage dependent \nSENSe<cnum>:IF:FILTer:STAGE<n>:COUNt? [char] \n(Read-only) Returns the number of taps in the digital filter of the specified stage. The filter sample \ncount setting is only used when SENSe:IF:FILTer:AUTO is set to False (MANUAL). \nCritical Note \nParameters \n<cnum> Existing channel number. If unspecified, <cnum> is set to 1. \n<n> Stage number. Choose 1 or 2 \n[char] Optional parameter. Choose from: \nnot specified - returns the current number of coefficients for the specified \nstage. \nMIN - returns the minimum number of coefficients for the specified \nstage. Stage1: 10, Stage2: 1 \nMAX - returns the maximum number of coefficients for the specified \nstage. Stage1 & 2: 1024 \nExamples SENS:IF:FILT:STAG2:COUN? \nsense2:if:filter:stage1:count? max \nReturn Type Numeric \nDefault Stage dependent \n1756\n\nSENSe<cnum>:IF:FILTer:STAGE1:FREQuency <value> \n(Read-Write) Sets and returns the Numerically Controlled Oscillator (NCO) frequency. This command \nis only used when SENSe:IF:FILTer:AUTO is set to False (Manual). \nCritical Note \nParameters \n<cnum> Existing channel number. If unspecified, <cnum> is set to 1. \n<value> Stage 1 Frequency. Min value= 0 Hz, Max value= 15 MHz. Or \nprogrammatically use the Max and Min queries to determine the range of \nsettable values. \nExamples SENS:IF:FILT:STAGe1:FREQ 9e6 \nsense2:if:filter:stage1:frequency 9.2e6 \nQuery Syntax SENSe<cnum>:IF:FILTer:STAGE1:FREQuency? \n'returns the current parameter value \nSENSe<cnum>:IF:FILTer:STAGE1:FREQuency? Min \n'returns the minimum frequency value. \nSENSe<cnum>:IF:FILTer:STAGE1:FREQuency? Max \n'returns the maximum frequency value. \nReturn Type Numeric \nDefault 9 MHz \nSENSe<cnum>:IF:FILTer:STAGE3:CATalog? \n(Read-only) Returns a list of strings for the currently supported filter types that can be used for the \nstage 3 filter. This command is only used when SENSe:IF:FILTer:AUTO is set to False (Manual). See \nSENS:IF:FILT:STAGe3:TYPE for a list of currently supported filter types. \nCritical Note \nParameters \n<cnum> Existing channel number. If unspecified, <cnum> is set to 1. \nExamples SENS:IF:FILT:STAGe3:CAT? \nsense2:if:filter:stage3:catalog? \nReturn Type String array \nDefault Not Applicable \n1757\n\nSENSe<cnum>:IF:FILTer:STAGe3:TYPE <value> \n(Read-Write) Sets and returns the Stage 3 filter type. This command is only used when \nSENSe:IF:FILTer:AUTO is set to False (Manual). \nCritical Note \nParameters \n<cnum> Existing channel number. If unspecified, <cnum> is set to 1. \n<value> (String) Filter type. Chose from: \n\"RECT\" Rectangular Window Filter \n\"TUKEY\" Tukey Filter \n\"PWIN\" Pulse Window Filter \nExamples SENS:IF:FILT:STAGe3:TYPE RECT \nsense2:if:filter:stage3:type pwin \nQuery Syntax SENSe<cnum>:IF:FILTer:STAGE3:TYPE? \nReturn Type String \nDefault \"TUKEY\" \nSENSe<cnum>:IF:FILTer:STAGe3:PARameter <p>, <value> \n(Read-Write) Sets and returns the Stage 3 filter parameters. \nMust first select the filter type (SENS:IF:FILT:STAGe3:TYPE) before setting these parameters \nUse SENSe:IF:FILT:STAGE3:PCAT? to return a list of the available parameters for the currently \nselected filter type. \nCritical Note \nParameters \n<cnum> Existing channel number. If unspecified, <cnum> is set to 1. \n<p> (String) Filter parameter. Choose from: \n\"C\" - Tap count (Tukey, RECT, PWIN) \n\"P\" - Period (PWIN ONLY) \n\"D\" - Delay (PWIN ONLY) \n\"W\" - Width (PWIN ONLY) \n\"R\" - Ramp
